vi "Select Server.vi"(8 "error in (no error)":errorcluster) -> (0 "error out":errorcluster, 3 "Selected Database":string)   [LabVIEW 2017]
panel:
  in  "Select":bool
  in  "DataBase List":i32(listbox)
  out "Database List":string[](array[string])
  # "SELECT SERVER"
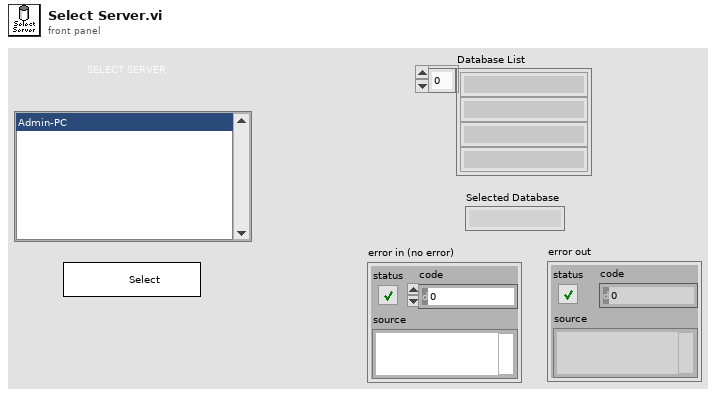
[diagram p1: front panel]
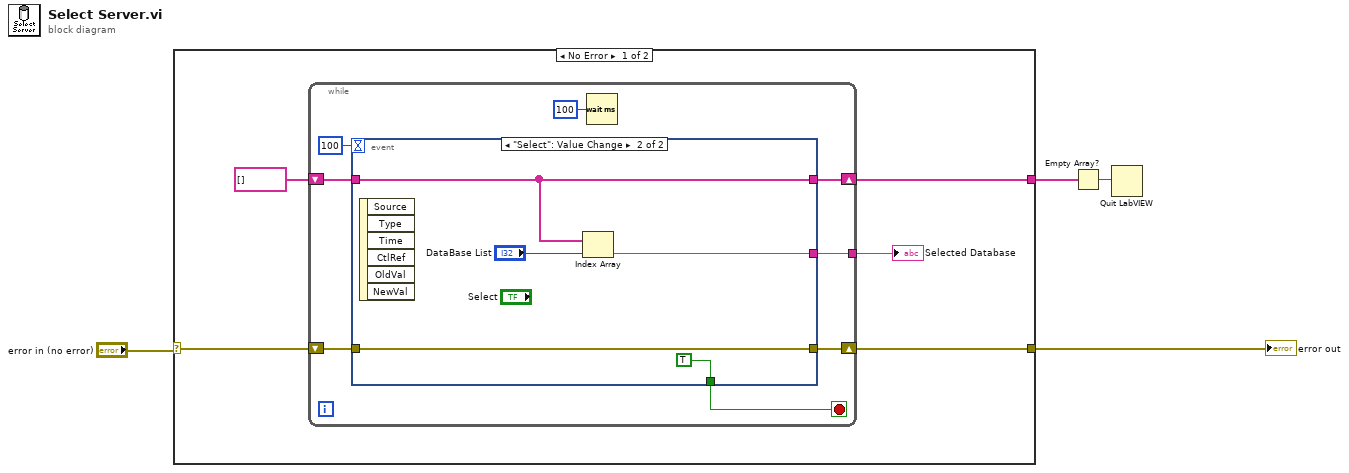
[diagram p0: block diagram]
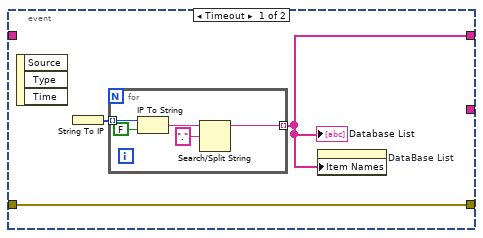
[diagram p2: hidden frame]
diagram:
  n1 = case shown="No Error" "error in (no error)" {
    selector: "error in (no error)" -> [w7 w31]
    tunnel: [w6 w31] -> w3
    tunnel: [w5 _] -> w2
    frame No Error {
      n2 = while {
        shift-right: [w16] -> w5
        shift-left: string[] [] -> [w15]
        tunnel: [w14] -> w8
        shift-right: [w10] -> w6
        shift-left: w7 -> [w11]
        stop <- w13 stop-if-true
        n3 = event shown="[1] \"Select\": Value Change" {
          selector: _ -> [_ _]
          dyn-events: _ -> [_ _]
          timeout: 100 -> [_ _]
          tunnel: [w19 w29] -> w16
          tunnel: w15 -> [_ w29]
          tunnel: [_ w28] -> w14
          tunnel: [_ TRUE] -> w13
          tunnel: w11 -> [w18 w26]
          tunnel: [w18 w26] -> w10
          event Timeout {
            n4 = event-data() -> ()  [unwired: 1 in, 3 out]
            n5 = String To IP() -> (0:w20:u32[])  [unwired: 1 in]
            n6 = for {
              tunnel: w20 -> [w25] mode=indexing
              tunnel: [w21] -> w19 mode=indexing
              n7 = IP To String(1:FALSE ("dot notation? (F)"), 2:w25) -> (0:w23:string)
              n8 = Search/Split String(string=w23, search string/char (-)="." ("regular expression")) -> (substring before match=w21:string)  [unwired: 1 in, 2 out]
            }
            "Database List" <- w19
            n9 = property on="DataBase List" class="LstBox (strict)"("Item Names"=w19) -> ()  [unwired: 2 in, 2 out]
          }
          event "Select": Value Change {
            n10 = event-data() -> ()  [unwired: 1 in, 6 out]
            n11 = Index Array(array=w29, index="DataBase List") -> (element=w28:string)
          }
        }
        n12 = Wait (ms)(milliseconds to wait=u32 100) -> ()  [unwired: 1 out]
      }
      "Selected Database" <- w8
    }
    frame Error {
    }
  }
  "error out" <- w3
  n13 = Empty Array?(array=w2) -> (empty?=w1:bool)
  n14 = Quit LabVIEW(quit? (T)=w1) -> ()
